vi "tcp发送.vi"(6 "写入缓冲区":string, 7 "命令":string(combo), 8 "error in (no error)":errorcluster caption="错误输入（无错误）", 10 "PORT":string, 11 "IP":string) -> (0 "错误输出":errorcluster, 3 "连接ID":refnum<k5>, 4 "读取缓冲区":string)   [LabVIEW 2016, in "数据传输系统-04.lvlib"]
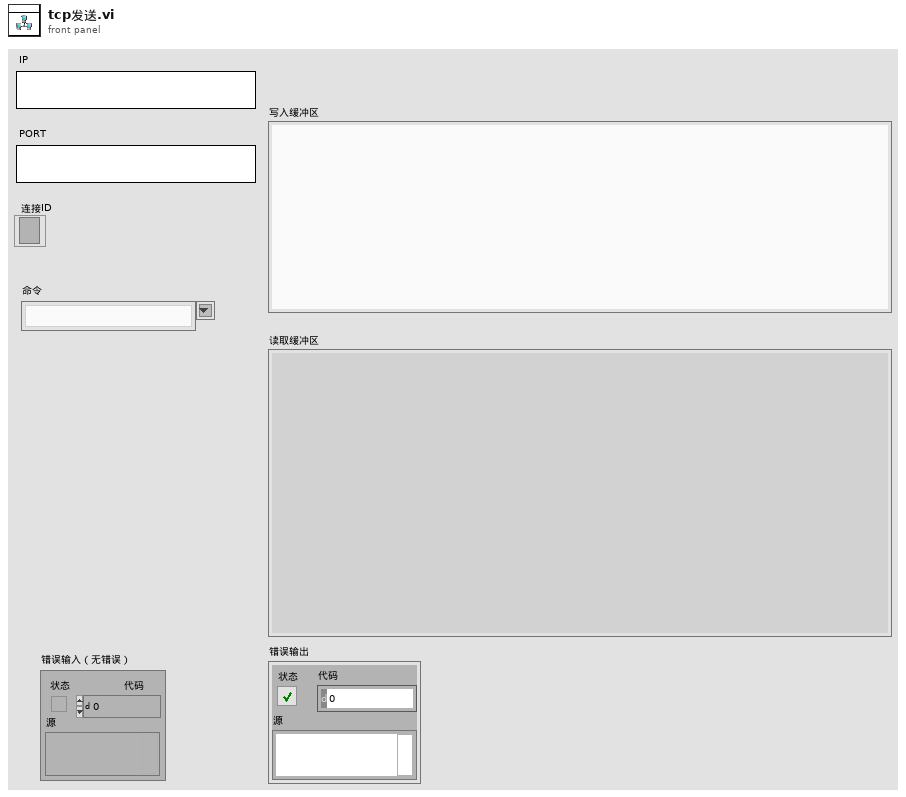
[diagram p1: front panel]
types:
  T1 = enum16{"Standard", "Buffered", "CRLF", "Immediate"}
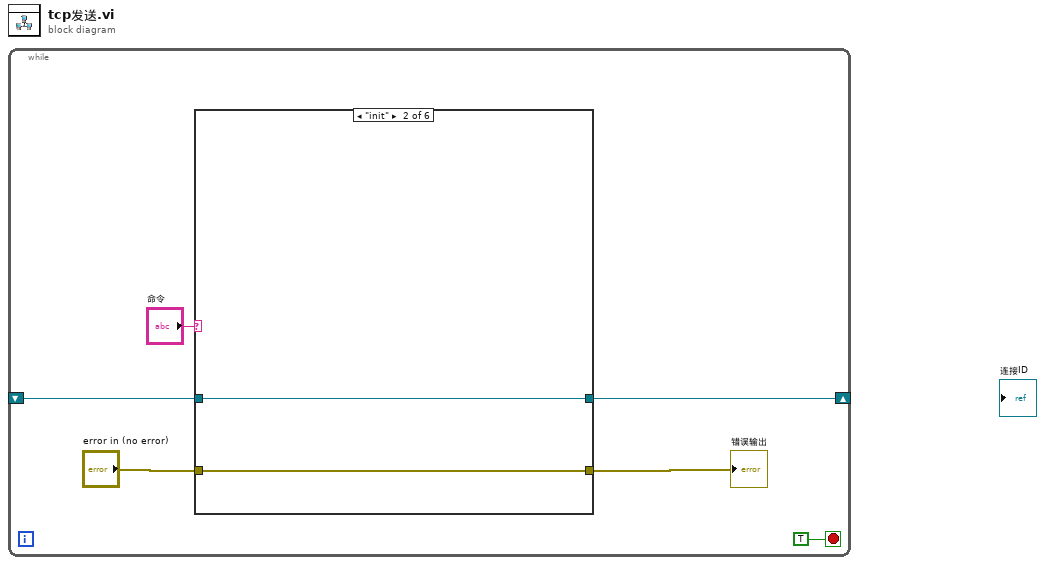
[diagram p0: block diagram]
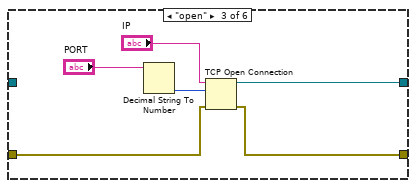
[diagram p3: hidden frame]
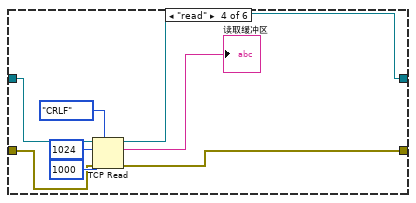
[diagram p4: hidden frame]
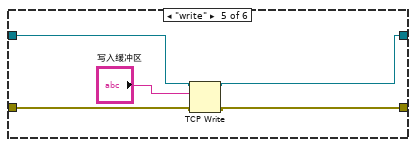
[diagram p5: hidden frame]
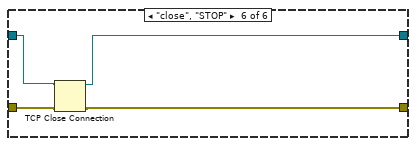
[diagram p6: hidden frame]
diagram:
  n1 = while {
    shift-right: [w3] -> _
    shift-left: _ -> [w1]
    stop <- TRUE stop-if-true
    n2 = case shown="\"init\"" "命令" {
      tunnel: "error in (no error)" -> [w8 w10 w12 w21 w27 w32]
      tunnel: [w8 w10 w11 w20 w26 w31] -> w5
      tunnel: w1 -> [w7 w9 _ w24 w29 w33]
      tunnel: [w7 w9 w13 w19 w25 w30] -> w3
      frame "idle", Default {
      }
      frame "init" {
      }
      frame "open" {
        n3 = Decimal String To Number(string="PORT") -> (number=w16:i32)  [unwired: 2 in, 1 out]
        n4 = TCP Open Connection(address="IP", remote port or service name=w16, error in (no error)=w12) -> (connection ID=w13:refnum<k5>, error out=w11:errorcluster)  [unwired: 2 in]
      }
      frame "read" {
        n5 = TCP Read(connection ID=w24, bytes to read=1024 ("读取的字节"), error in (no error)=w21, 7:T1."CRLF" ("模式（标准）"), 9:1000 ("超时毫秒(25000)")) -> (connection ID out=w19:refnum<k5>, data out=→"读取缓冲区":string, error out=w20:errorcluster)
      }
      frame "write" {
        n6 = TCP Write(connection ID=w29, data in="写入缓冲区", error in (no error)=w27) -> (connection ID out=w25:refnum<k5>, error out=w26:errorcluster)  [unwired: 1 in, 1 out]
      }
      frame "close", "STOP" {
        n7 = TCP Close Connection(connection ID=w33, error in (no error)=w32) -> (connection ID out=w30:refnum<k5>, error out=w31:errorcluster)  [unwired: 1 in]
      }
    }
    "错误输出" <- w5
  }
